vi "Create New File.vi"(6 "Scanner 2?  (Scanner1)":bool, 8 "error in (no error)":errorcluster, 10 "Scanner 1":refnum<file>, 11 "Scanner 2":refnum<file>) -> (0 "error out":errorcluster, 2 "Scanner 1 File out":refnum<file>, 3 "Scanner 2 File out":refnum<file>)   [LabVIEW 2013]
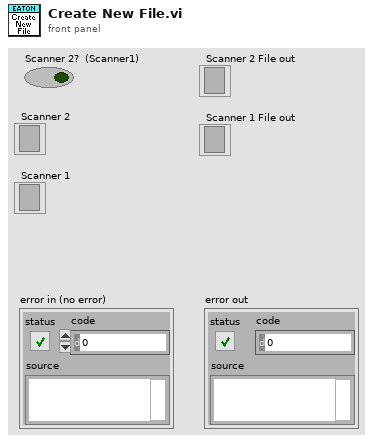
[diagram p1: front panel]
types:
  T1 = enum16{"open", "replace", "create", "open or create", "replace or create", "replace or create with confirmation"}
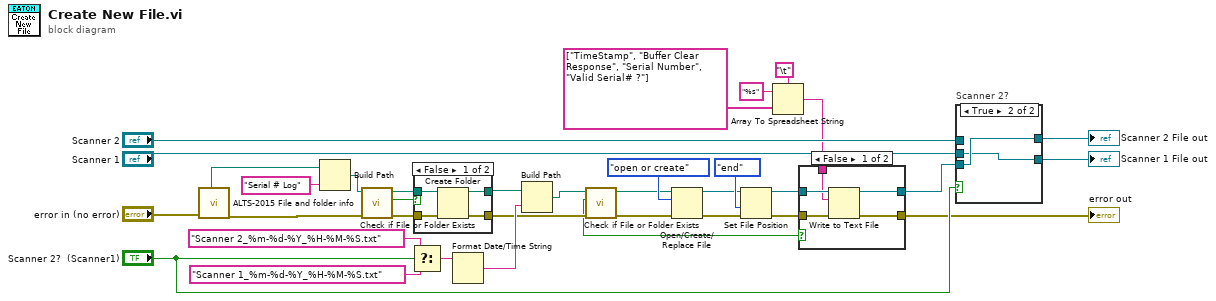
[diagram p0: block diagram]
diagram:
  n1 = call "ALTS-2015 File and folder info.vi"("error in (no error)"="error in (no error)") -> ("Info Folder"=w1:path, "error out"=w23:errorcluster)  [unwired: 9 in, 8 out]
  n2 = Build Path(base path=w1, name or relative path="Serial # Log") -> (appended path=w24:path)
  n3 = call <vilib>:"Check if File or Folder Exists.vi"("error in (no error)"=w23, "path"=w24) -> ("error out"=w10:errorcluster, "file or folder exists?"=w12:bool, "dup path"=w11:path)  [unwired: 7 in]
  n4 = Select(t="Scanner 2_%m-%d-%Y_%H-%M-%S.txt" ("time format string (%c)"), s="Scanner 2?  (Scanner1)", f="Scanner 1_%m-%d-%Y_%H-%M-%S.txt" ("time format string (%c)")) -> (s? t:f=w29:string)
  n5 = case shown="False" w12 {
    tunnel: w11 -> [w39 w41]
    tunnel: w10 -> [w38 w40]
    tunnel: [w37 w41] -> w9
    tunnel: [w36 w40] -> w21
    frame False {
      n6 = Create Folder(path (use dialog)=w39, error in=w38) -> (created path=w37:path, error out=w36:errorcluster)  [unwired: 1 in, 1 out]
    }
    frame True {
    }
  }
  n7 = Format Date/Time String(time format string (%c)=w29) -> (date/time string=w26:string)  [unwired: 2 in]
  n8 = Build Path(base path=w9, name or relative path=w26) -> (appended path=w4:path)
  n9 = call <vilib>:"Check if File or Folder Exists.vi"("error in (no error)"=w21, "path"=w4) -> ("error out"=w5:errorcluster, "file or folder exists?"=w2:bool, "dup path"=w3:path)  [unwired: 7 in]
  n10 = Open/Create/Replace File(file path (use dialog)=w3, error in=w5, operation (0:open)=T1."open or create") -> (refnum out=w7:refnum<file>, error out=w8:errorcluster)  [unwired: 3 in, 1 out]
  n11 = Set File Position(refnum=w7, from (0:start)=enum16{"start", "end", "current"}."end", error in=w8) -> (refnum out=w19:refnum<file>, error out=w20:errorcluster)  [unwired: 1 in]
  n12 = Array To Spreadsheet String(delimiter (Tab)="\t", array=string[] ["TimeStamp", "Buffer Clear Response", "Serial Number", "Valid Serial# ?"] ("Write Text"), 3:"%s" ("format string")) -> (spreadsheet string=w17:string)
  n13 = case shown="False" w2 {
    tunnel: [w46 w48] -> w31
    tunnel: w20 -> [w45 w47]
    tunnel: w19 -> [w44 w48]
    tunnel: [w43 w47] -> w18
    tunnel: w17 -> [w42 _]
    frame False {
      n14 = Write to Text File(file (use dialog)=w44, text=w42, error in=w45) -> (refnum out=w46:refnum<file>, error out=w43:errorcluster)  [unwired: 1 in, 1 out]
    }
    frame True {
    }
  }
  "error out" <- w18
  n15 = case "Scanner 2?" shown="True" "Scanner 2?  (Scanner1)" {
    tunnel: [w49 w52] -> w32
    tunnel: w31 -> [w50 w52]
    tunnel: "Scanner 2" -> [w49 _]
    tunnel: "Scanner 1" -> [_ w51]
    tunnel: [w50 w51] -> w35
    frame False {
    }
    frame True {
    }
  }
  "Scanner 1 File out" <- w35
  "Scanner 2 File out" <- w32
